vi "PulseTrain-Create (Continuous PBP).vi"(0 "State In":T1, 5 "Pulse Rate (Hz)":dbl=1.0 min=1.0 max=40.0, 7 "Phase (cycles)":dbl=1.0 min=1.0 max=40.0, 9 "Fs (Hz)":dbl, 11 "Npts":i32) -> (4 "State Out":T1, 8 "Buffer":dbl[](array[numeric]), 15 "New period?":bool)   [LabVIEW 2020]
uses:
  PT-Continuous State.ctl
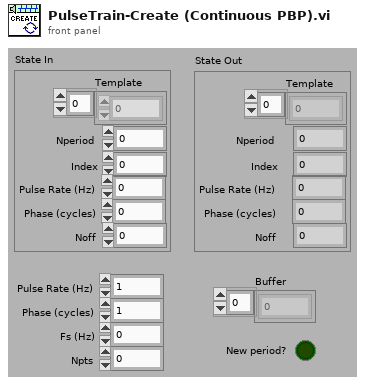
[diagram p1: front panel]
types:
  T1 = typedef "PT-Continuous State.ctl" = cluster{"Template":dbl[], "Nperiod":i32, "Index":i32, "Pulse Rate (Hz)":dbl, "Phase (cycles)":dbl, "Noff":i32}
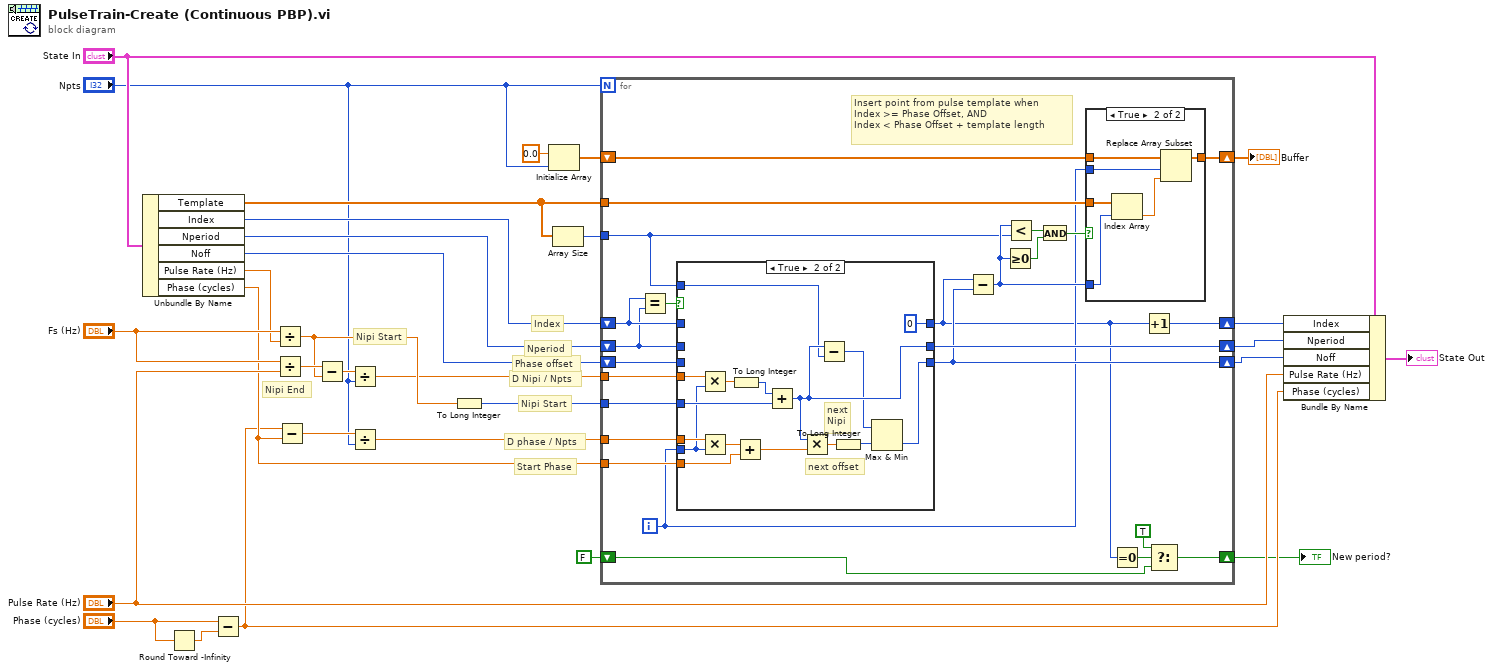
[diagram p0: block diagram]
diagram:
  # "Nperiod"
  # "Index"
  # "Start Phase"
  # "Phase offset"
  # "Nipi Start"
  # "D phase / Npts"
  # "D Nipi / Npts"
  # "Nipi End"
  # "Nipi Start"
  n1 = Unbundle By Name("State In") -> ("Template"=w12:dbl[], "Index"=w16:i32, "Nperiod"=w13:i32, "Noff"=w15:i32, "Pulse Rate (Hz)"=w25:dbl, "Phase (cycles)"=w17:dbl)
  n2 = Round Toward -Infinity(1:"Phase (cycles)") -> (0:w4:dbl)
  n3 = Subtract(x="Phase (cycles)", y=w4) -> (x-y=w5:dbl)
  n4 = Divide(x="Fs (Hz)", y=w25) -> (x/y=w22:dbl)
  n5 = Divide(x="Fs (Hz)", y="Pulse Rate (Hz)") -> (x/y=w23:dbl)
  n6 = Subtract(x=w5, y=w17) -> (x-y=w19:dbl)
  n7 = Subtract(x=w23, y=w22) -> (x-y=w21:dbl)
  n8 = Divide(x=w21, y="Npts") -> (x/y=w20:dbl)
  n9 = Divide(x=w19, y="Npts") -> (x/y=w18:dbl)
  n10 = To Long Integer(number=w22) -> (32bit integer=w24:i32)
  n11 = Initialize Array(0.0 ("element"), "Npts") -> (w14:dbl[])
  n12 = Array Size(array=w12) -> (size(s)=w11:i32)
  n13 = for {
    N: "Npts" -> [_]
    tunnel: w12 -> [w40]
    shift-right: [w46] -> w9
    shift-left: w16 -> [w51]
    tunnel: w24 -> [w55]
    tunnel: w20 -> [w54]
    tunnel: w18 -> [w53]
    shift-right: [w45] -> w7
    shift-left: w15 -> [w47]
    tunnel: w17 -> [w52]
    shift-right: [w49] -> w8
    shift-left: w13 -> [w48]
    tunnel: w11 -> [w36]
    shift-right: [w37] -> w10
    shift-left: w14 -> [w39]
    shift-right: [w33] -> w1
    shift-left: FALSE -> [w31]
    i -> [w38]
    # "Insert point from pulse template when \nIndex >= Phase Offset, AND\nIndex < Phase Offset + template length"
    n14 = Equal?(x=w51, y=w48) -> (x = y?=w50:bool)
    n15 = case shown="True" w50 {
      tunnel: w55 -> [_ w81]
      tunnel: w54 -> [_ w79]
      tunnel: w53 -> [_ w77]
      tunnel: [w64 w70] -> w49
      tunnel: w52 -> [_ w75]
      tunnel: [w63 w66] -> w45
      tunnel: w51 -> [w65 _]
      tunnel: [w65 0 ("Index")] -> w34
      tunnel: w48 -> [w64 _]
      tunnel: w47 -> [w63 _]
      tunnel: w38 -> [_ w73]
      tunnel: w36 -> [_ w69]
      frame False {
      }
      frame True {
        # "next offset"
        # "next\nNipi"
        n16 = Multiply(x=w79, y=w73) -> (x*y=w80:dbl)
        n17 = Multiply(x=w77, y=w73) -> (x*y=w76:dbl)
        n18 = To Long Integer(number=w80) -> (32bit integer=w78:i32)
        n19 = Add(x=w76, y=w75) -> (x+y=w72:dbl)
        n20 = Add(x=w78, y=w81) -> (x+y=w70:i32)
        n21 = Multiply(x=w70, y=w72) -> (x*y=w71:dbl)
        n22 = Subtract(x=w70, y=w69) -> (x-y=w68:i32)
        n23 = To Long Integer(number=w71) -> (32bit integer=w67:i32)
        n24 = Max & Min(x=w68, y=w67) -> (min(x,y)=w66:i32)  [unwired: 1 out]
      }
    }
    n25 = Subtract(x=w34, y=w45) -> (x-y=w41:i32)
    n26 = Greater Or Equal To 0?(x=w41) -> (x >= 0?=w43:bool)
    n27 = Less?(x=w41, y=w36) -> (x < y?=w44:bool)
    n28 = And(x=w44, y=w43) -> (x .and. y?=w42:bool)
    n29 = case shown="True" w42 {
      tunnel: w41 -> [_ w61]
      tunnel: w40 -> [_ w62]
      tunnel: w39 -> [w56 w60]
      tunnel: w38 -> [_ w58]
      tunnel: [w56 w57] -> w37
      frame False {
      }
      frame True {
        n30 = Index Array(array=w62, index=w61) -> (element=w59:dbl)
        n31 = Replace Array Subset(array=w60, new element=w59, index=w58) -> (w57:dbl[])
      }
    }
    n32 = Equal To 0?(x=w34) -> (x = 0?=w35:bool)
    n33 = Increment(x=w34) -> (x+1=w46:i32)
    n34 = Select(t=TRUE, s=w35, f=w31) -> (s? t:f=w33:bool)
  }
  "Buffer" <- w10
  "New period?" <- w1
  n35 = Bundle By Name(cluster="State In", "Index"=w9, "Nperiod"=w8, "Noff"=w7, "Pulse Rate (Hz)"="Pulse Rate (Hz)", "Phase (cycles)"=w5) -> (→"State Out":T1)
